vi "Configure Channel (GS Scale).vi"(0 "VISA resource name":refnum<visa-resource-name>, 1 "Scaling":T2={"Floating point position (2)"=2, "Lower Scaling (0)"=0.0, "Upper Scaling (100.00)"=100.0, "Unit Character (\"\")"=""} {"Upper Scaling (100.00)" format="%_6g"; "Lower Scaling (0)" format="%_6g"; "Floating point position (2)" min=0 max=5 step=1}, 2 "Low cut":T1={"Enable Low-cut Filter (False)"=FALSE, "Low-cut (5)"=5.0} {"Low-cut (5)" min=0.0 max=5.0 format="%.1f"}, 5 "Channel (0001)":string="0001", 7 "Enable Channel (True)":bool=TRUE, 9 "Range, Span, Bias":T3={"GS Range (0 : 1-5V)"=0, "Enable Span (False)"=FALSE, "Lower Span (-2.0000)"=-2.0, "Upper Span (2.0000)"=2.0, "Bias (0)"=0.0} {"Upper Span (2.0000)" min=-99999.0 max=99999.0 step=1.0 format="%_5g"; "Lower Span (-2.0000)" min=-99999.0 max=99999.0 step=1.0 format="%_5g"; "GS Range (0 : 1-5V)" items=["1-5V", "0.4-2V"]}, 11 "error in (no error)":errorcluster) -> (4 "VISA resource name out":refnum<visa-resource-name>, 6 "Channel":string, 15 "error out":errorcluster)   [LabVIEW 2020, in "Yokogawa GX Series.lvlib"]
doc: "Sets the input range as GS.\n\nCommand: SRangeAI"
uses:
  <instrlib>/Yokogawa GX Series/Yokogawa GX Series.lvlib
  <instrlib>/Yokogawa GX Series/Private/GS Range.vi
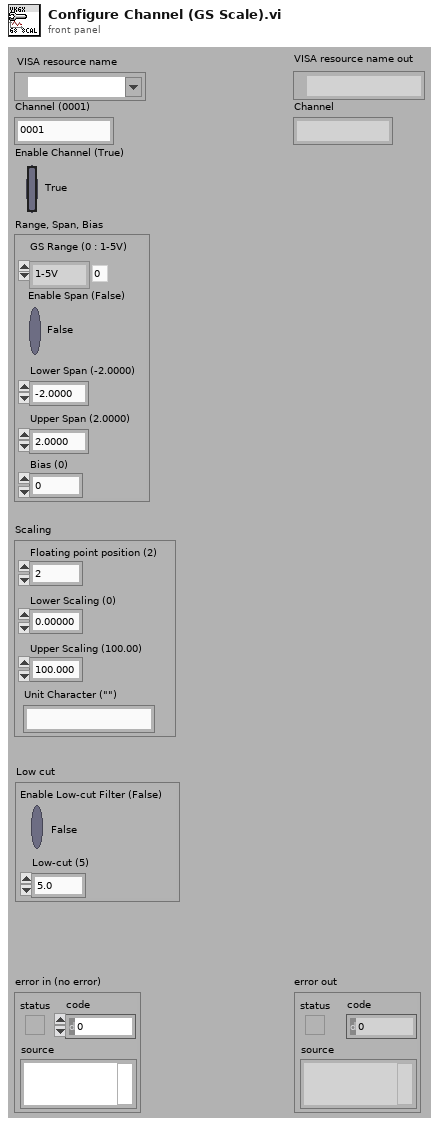
[diagram p1: front panel]
types:
  T1 = cluster{"Enable Low-cut Filter (False)":bool, "Low-cut (5)":dbl}
  T2 = cluster{"Floating point position (2)":i32, "Lower Scaling (0)":dbl, "Upper Scaling (100.00)":dbl, "Unit Character (\"\")":string}
  T3 = cluster{"GS Range (0 : 1-5V)":i32, "Enable Span (False)":bool, "Lower Span (-2.0000)":dbl, "Upper Span (2.0000)":dbl, "Bias (0)":dbl}
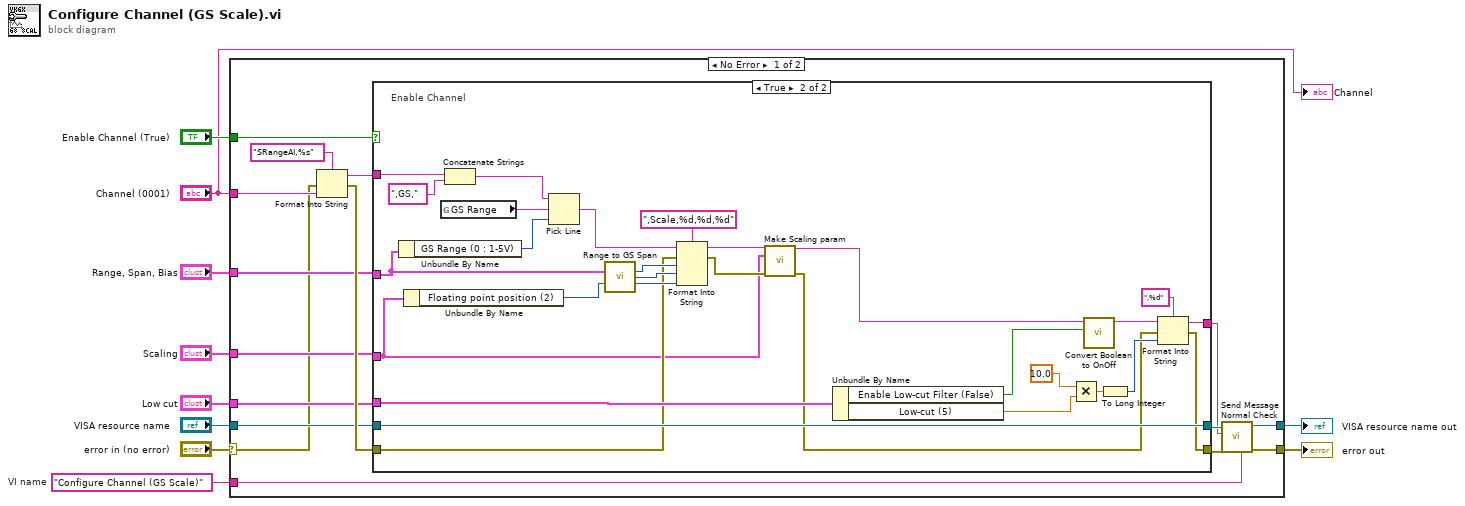
[diagram p0: block diagram]
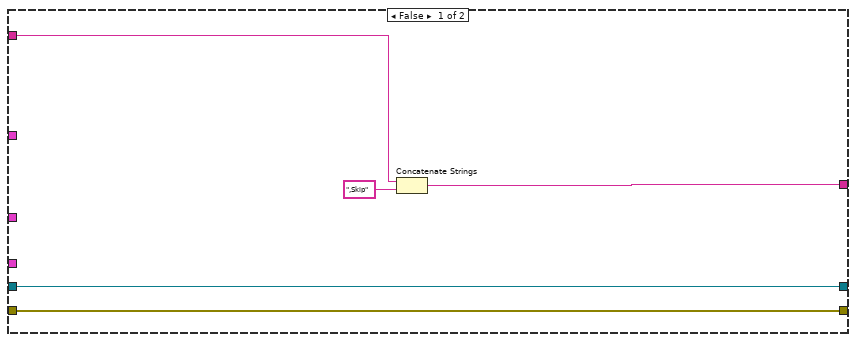
[diagram p2: hidden frame]
diagram:
  w3 = "Configure Channel (GS Scale)"  # VI name
  n1 = case shown="No Error" "error in (no error)" {
    selector: "error in (no error)" -> [w11 w61]
    tunnel: "Enable Channel (True)" -> [w23 _]
    tunnel: "VISA resource name" -> [w22 w62]
    tunnel: "Range, Span, Bias" -> [w21 _]
    tunnel: "Scaling" -> [w20 _]
    tunnel: "Low cut" -> [w19 _]
    tunnel: [w17 w62] -> w5
    tunnel: [w16 w61] -> w4
    tunnel: w3 -> [w14 _]
    tunnel: "Channel (0001)" -> [w12 _]
    frame No Error {
      n2 = Format Into String(format string="SRangeAI,%s", error in=w11, w12) -> (resulting string=w24:string, error out=w25:errorcluster)  [unwired: 1 in]
      n3 = case shown="True" w23 {
        tunnel: w25 -> [w28 w49]
        tunnel: [w28 w44] -> w13
        tunnel: w24 -> [w29 w59]
        tunnel: [w31 w45] -> w15
        tunnel: w22 -> [w27 w50]
        tunnel: [w27 w50] -> w18
        tunnel: w21 -> [_ w57]
        tunnel: w20 -> [_ w37]
        tunnel: w19 -> [_ w51]
        frame False {
          n4 = Concatenate Strings(w29, ",Skip") -> (w31:string)
        }
        frame True {
          # "Enable Channel"
          n5 = Unbundle By Name(w57) -> ("GS Range (0 : 1-5V)"=w56:i32)
          n6 = Unbundle By Name(w37) -> ("Floating point position (2)"=w40:i32)
          n7 = global read "GS Range.vi" "GS Range"() -> (w32:string)
          n8 = Concatenate Strings(w59, ",GS,") -> (w58:string)
          n9 = Pick Line(string ("")=w58, multi-line string=w32, line index=w56) -> (output string=w48:string)
          n10 = call <instrlib>:"Range to GS Span.vi"("Range and span"=w57, "Floating Point Position (2)"=w40) -> ("Lower Span"=w54:i32, "Upper Span"=w53:i32, "Bias"=w52:i32)  [unwired: 11 in]
          n11 = Format Into String(format string=",Scale,%d,%d,%d", initial string=w48, error in=w49, w54, w53, w52) -> (resulting string=w39:string, error out=w38:errorcluster)
          n12 = call <instrlib>:"Make Scaling param.vi"("String (\"\")"=w39, "Scaling"=w37, "error in (no error)"=w38) -> ("String After"=w36:string, "error out"=w33:errorcluster)  [unwired: 11 in]
          n13 = Unbundle By Name(w51) -> ("Enable Low-cut Filter (False)"=w35:bool, "Low-cut (5)"=w34:dbl)
          n14 = Multiply(x=10.0, y=w34) -> (x*y=w42:dbl)
          n15 = call <instrlib>:"Convert Boolean to OnOff.vi"("On/Off"=w35, "Initial String (\"\")"=w36) -> ("Resulting String"=w47:string)  [unwired: 9 in]
          n16 = To Long Integer(number=w42) -> (32bit integer=w41:i32)
          n17 = Format Into String(format string=",%d", initial string=w47, error in=w33, w41) -> (resulting string=w45:string, error out=w44:errorcluster)
        }
      }
      n18 = call <instrlib>:"Send Message Normal Check.vi"("Source (\"\")"=w14, "error in (no error)"=w13, "Send Message (\"\")"=w15, "VISA resource name"=w18) -> ("error out"=w16:errorcluster, "VISA resource name out"=w17:refnum<visa-resource-name>)  [unwired: 2 in, 4 out]
    }
    frame Error {
    }
  }
  "error out" <- w4
  "VISA resource name out" <- w5
  "Channel" <- "Channel (0001)"
